vi "Heater Range Calc.vi"(2 "Power":dbl format="%.2e", 3 "Heater Range":u32, 4 "Start Control?":bool, 5 "Resistance":dbl format="%.2f") -> (0 "Command":string, 1 "Heater Range Out":u32)   [LabVIEW 2020]
panel:
  out "Max Range power":dbl format="%.2e"
  out "Range":dbl format="%.2e"
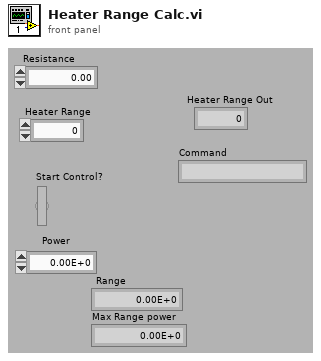
[diagram p1: front panel]
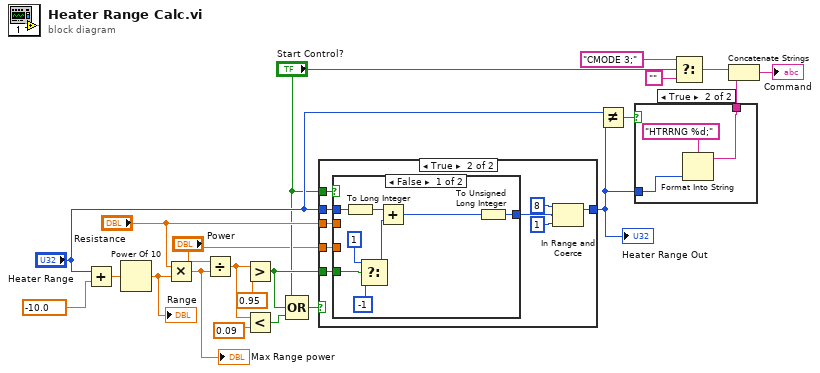
[diagram p0: block diagram]
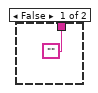
[diagram p2: hidden frame]
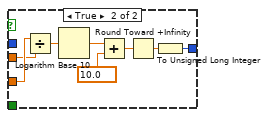
[diagram p4: hidden frame]
diagram:
  n1 = Add(x="Heater Range", y=-10.0) -> (x+y=w5:dbl)
  n2 = Power Of 10(x=w5) -> (10^x=w4:dbl)
  "Range" <- w4
  n3 = Multiply(x="Resistance", y=w4) -> (x*y=w1:dbl)
  "Max Range power" <- w1
  n4 = Divide(x="Power", y=w1) -> (x/y=w17:dbl)
  n5 = Greater?(x=w17, y=0.95) -> (0:w11:bool)
  n6 = Less?(x=w17, y=0.09) -> (x < y?=w13:bool)
  n7 = Compound Arithmetic op=OR("Start Control?", w11, w13) -> (w14:bool)
  n8 = case shown="True" w14 {
    tunnel: "Heater Range" -> [w22 w28]
    tunnel: [w22 w27] -> w8
    tunnel: w11 -> [_ w31]
    tunnel: "Power" -> [_ w25]
    tunnel: "Resistance" -> [_ w24]
    tunnel: "Start Control?" -> [_ w23]
    frame False {
    }
    frame True {
      n9 = case shown="False" w23 {
        tunnel: w31 -> [w39 _]
        tunnel: w28 -> [w36 _]
        tunnel: [w32 w43] -> w26
        tunnel: w25 -> [_ w45]
        tunnel: w24 -> [_ w44]
        frame False {
          n10 = To Long Integer(number=w36) -> (32bit integer=w33:i32)
          n11 = Select(t=1 ("Heater Range"), s=w39, f=-1) -> (s? t:f=w35:i32)
          n12 = Add(x=w33, y=w35) -> (x+y=w34:i32)
          n13 = To Unsigned Long Integer(number=w34) -> (unsigned 32bit integer=w32:u32)
        }
        frame True {
          n14 = Divide(x=w45, y=w44) -> (x/y=w41:dbl)
          n15 = Logarithm Base 10(1:w41) -> (0:w42:dbl)
          n16 = Add(x=w42, y=10.0) -> (x+y=w40:dbl)
          n17 = Round Toward +Infinity(x=w40) -> (ceil(x): smallest int >= x=w46:dbl)
          n18 = To Unsigned Long Integer(number=w46) -> (unsigned 32bit integer=w43:u32)
        }
      }
      n19 = In Range and Coerce(upper limit=u32 8, x=w26, lower limit=u32 1) -> (coerced(x)=w27:u32)  [unwired: 1 out]
    }
  }
  "Heater Range Out" <- w8
  n20 = Not Equal?(x="Heater Range", y=w8) -> (x != y?=w10:bool)
  n21 = case shown="True" w10 {
    tunnel: ["" w49] -> w9
    tunnel: w8 -> [_ w51]
    frame False {
    }
    frame True {
      n22 = Format Into String(format string="HTRRNG %d;", w51) -> (resulting string=w49:string)  [unwired: 2 in, 1 out]
    }
  }
  n23 = Select(t="CMODE 3;", s="Start Control?", f="") -> (s? t:f=w19:string)
  n24 = Concatenate Strings(w19, w9) -> (→"Command":string)
